vi "Compiled.Get Data Settings.vi"(6 "Cluster":refnum<k21>, 8 "error in (no error)":errorcluster, 9 "Node.Settings":T3 {"Name" format="%.0x"}, 10 "Node Ref in":T1 format="%.0x", 11 "Addon Ref In":T1 format="%.0x") -> (0 "error out":errorcluster, 1 "Node Data Refs":T4 {"Outgoing"."Trigger.Refs"."Data Reference" format="%.0x"; "Outgoing"."Disable.Refs"."Data Reference" format="%.0x"; "Outgoing"."Data.Refs"."Data Reference" format="%.0x"; "Incoming"."Timing.Refs"."Data Reference" format="%.0x"; "Incoming"."Data.Refs"."Data Reference" format="%.0x"}, 2 "Node Ref out":T1 format="%.0x", 3 "Addon Ref out":T1 format="%.0x", 4 "Async Refs":T2(array[cluster]) {"VS Refs" format="%.0x"})   [LabVIEW 2015, in "J1939 Addon System Explorer.lvlib"]
uses:
  J1939 Addon System Explorer.lvlib
  Shared/Types/Device Settings.ctl
  Shared/Types/Incoming Settings.ctl
  Shared/Types/Incoming Frame Settings.ctl
  <vilib>/NI Veristand/Custom Device API/Block Data Reference.ctl
  <vilib>/NI Veristand/Custom Device API/Data Reference.ctl
  Shared/Types/Outgoing Settings.ctl
  Shared/Types/Outgoing Frame Settings.ctl
  Shared/Types/Outgoing Event Trigger Types.ctl
  Protection Support/Source/Shared/Types/Exported Frame Settings.ctl
  Protection Support/Source/Shared/Types/Exported Frame Type.ctl
  Protection Support/Source/Shared/Types/Exported Protection Settings.ctl
  Protection Support/Source/Shared/Types/Protection Type.ctl
  Protection Support/Source/Shared/Types/XNET Signal Configuration.ctl
  Protection Support/Source/Shared/Types/Exported Counter Settings.ctl
  Protection Support/Source/Shared/Types/Exported Event Trigger Type.ctl
  <vilib>/NI Veristand/Custom Device API/Custom Device Item Ref.ctl
  Shared/Types/Monitor Settings.ctl
  <vilib>/NI Veristand/Custom Device API/Data Access Type.ctl
  Types/Compiled Refs.ctl
  Protection Support/Source/System Explorer/Types/Export Frame GUIDs List.ctl
  Protection Support/Source/System Explorer/Types/Export Frames List and Type.ctl
  Protection Support/Source/System Explorer/Types/Exported Frame Settings.ctl
  <vilib>/NI Veristand/Custom Device Tools/Custom Device Utility Library/NI VeriStand - Search for Item by GUID.vi
  Shared/SubVIs/Constants.vi
  <vilib>/NI VeriStand/Custom Device Tools/Custom Device Utility Library/Custom Device Utility Library.lvlib
  Shared/J1939 Addon Shared.lvlib
  <vilib>/NI VeriStand/Custom Device API/Custom Device API.lvlib
  Protection Support/Source/Shared/Protection and Counter Support Shared.lvlib
  Protection Support/Source/System Explorer/Protection and Counter Support System Explorer.lvlib
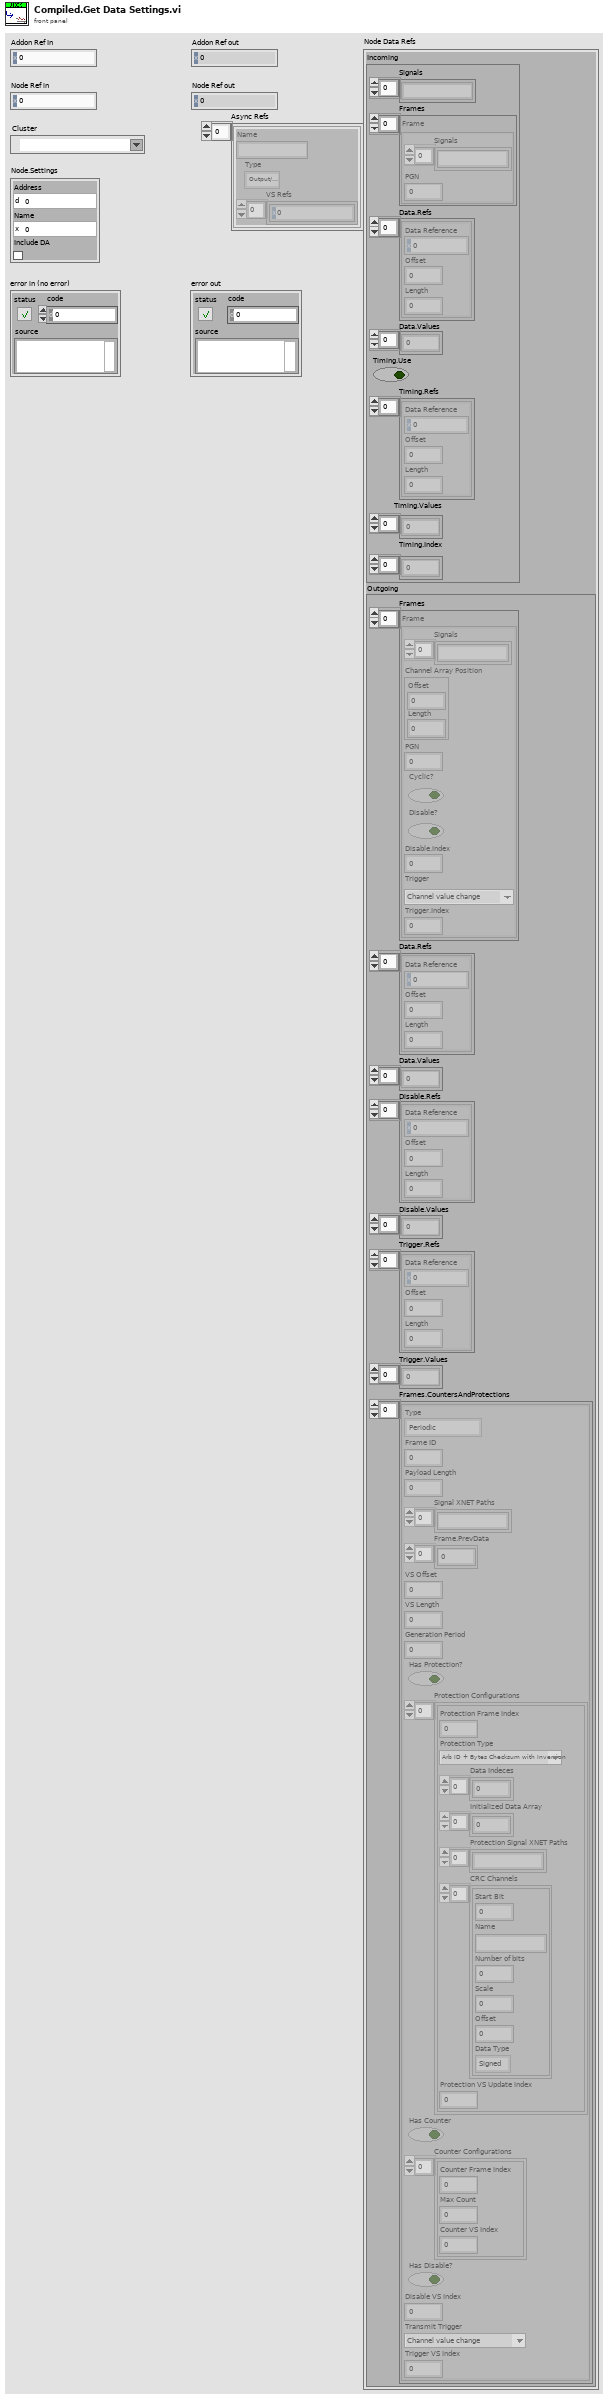
[diagram p1: front panel]
types:
  T1 = typedef "Custom Device API.lvlib/Custom Device Item Ref.ctl" = u64
  T2 = cluster{"Name":string, "Type":enum16{"Output/Write", "Input/Read", "Input/ReadWrite"}, "VS Refs":T1[]}[]
  T3 = typedef "J1939 Addon Shared.lvlib/Monitor Settings.ctl" = cluster{"Address":u8, "Name":u64, "Include DA":bool}
  T4 = typedef "J1939 Addon Shared.lvlib/Device Settings.ctl" = cluster{"Incoming":T5, "Outgoing":T9}
  T5 = typedef "J1939 Addon Shared.lvlib/Incoming Settings.ctl" = cluster{"Signals":string[], "Frames":T6[], "Data.Refs":T7[], "Data.Values":dbl[], "Timing.Use":bool, "Timing.Refs":T7[], "Timing.Values":dbl[], "Timing.Index":i32[]}
  T6 = typedef "J1939 Addon Shared.lvlib/Incoming Frame Settings.ctl" = cluster{"Signals":string[], "PGN":u32}
  T7 = typedef "Custom Device API.lvlib/Block Data Reference.ctl" = cluster{"Data Reference":T8, "Offset":u64, "Length":u64}
  T8 = typedef "Custom Device API.lvlib/Data Reference.ctl" = i32
  T9 = typedef "J1939 Addon Shared.lvlib/Outgoing Settings.ctl" = cluster{"Frames":T10[], "Data.Refs":T7[], "Data.Values":dbl[], "Disable.Refs":T7[], "Disable.Values":dbl[], "Trigger.Refs":T7[], "Trigger.Values":dbl[], "Frames.CountersAndProtections":T12[]}
  T10 = typedef "J1939 Addon Shared.lvlib/Outgoing Frame Settings.ctl" = cluster{"Signals":string[], "Channel Array Position":cluster{"Offset":u32, "Length":u32}, "PGN":u32, "Cyclic?":bool, "Disable?":bool, "Disable.Index":i32, "Trigger":T11, "Trigger.Index":i32}
  T11 = typedef "J1939 Addon Shared.lvlib/Outgoing Event Trigger Types.ctl" = enum16{"Channel value change", "Trigger channel (not zero)", "Channel value change or trigger channel (not zero)", "Trigger channel (any value change)", "Channel value change or trigger channel (any value change)"}
  T12 = typedef "Protection and Counter Support Shared.lvlib/Exported Frame Settings.ctl" = cluster{"Type":T13, "Frame ID":u32, "Payload Length":u32, "Signal XNET Paths":string[], "Frame.PrevData":dbl[], "VS Offset":i32, "VS Length":i32, "Generation Period":u32, "Has Protection?":bool, "Protection Configurations":T14[], "Has Counter":bool, "Counter Configurations":T17[], "Has Disable?":bool, "Disable VS Index":i32, "Transmit Trigger":T18, "Trigger VS Index":i32}
  T13 = typedef "Protection and Counter Support Shared.lvlib/Exported Frame Type.ctl" = enum16{"Periodic", "Event", "Periodic/Event"}
  T14 = typedef "Protection and Counter Support Shared.lvlib/Exported Protection Settings.ctl" = cluster{"Protection Frame Index":i32, "Protection Type":T15, "Data Indeces":i32[], "Initialized Data Array":dbl[], "Protection Signal XNET Paths":string[], "CRC Channels":T16[], "Protection VS Update Index":i32}
  T15 = typedef "Protection and Counter Support Shared.lvlib/Protection Type.ctl" = enum16{"Arb ID + Bytes Checksum with Inversion", "Arb ID + Bytes CRC with Inversion", "Reversed Raw Signal Checksum with Inversion"}
  T16 = typedef "Protection and Counter Support Shared.lvlib/XNET Signal Configuration.ctl" = cluster{"Start Bit":i32, "Name":string, "Number of bits":i32, "Scale":dbl, "Offset":dbl, "Data Type":u32}
  T17 = typedef "Protection and Counter Support Shared.lvlib/Exported Counter Settings.ctl" = cluster{"Counter Frame Index":i32, "Max Count":dbl, "Counter VS Index":i32}
  T18 = typedef "Protection and Counter Support Shared.lvlib/Exported Event Trigger Type.ctl" = enum16{"Channel value change", "Trigger channel (not zero)", "Channel value change or trigger channel (not zero)", "Trigger channel (any value change)", "Channel value change or trigger channel (any value change)"}
  T19 = cluster{"Name":string, "Type":enum16{"Output/Write", "Input/Read", "Input/ReadWrite"}, "VS Refs":T1[]}
  T20 = typedef "Protection and Counter Support System Explorer.lvlib/Export Frame GUIDs List.ctl" = cluster{"Signal Page GUID":string, "Rolling Counter Value GUID":string, "Protection Value GUID":string}
  T21 = typedef "J1939 Addon System Explorer.lvlib/Compiled Refs.ctl" = cluster{"VS Refs":T1[], "Disable Refs":T1[], "Trigger Refs":T1[]}
  T22 = typedef "Custom Device API.lvlib/Data Access Type.ctl" = enum16{"Read", "Write"}
  T23 = typedef "Protection and Counter Support System Explorer.lvlib/Export Frames List and Type.ctl" = cluster{"Type":T13, "Frame Refs":T1[], "Frame Settings":T24[]}
  T24 = typedef "Protection and Counter Support System Explorer.lvlib/Exported Frame Settings.ctl" = cluster{"ID":u32, "Disable Transmission":bool, "Disable Transmission Ref":T1, "Transmit Trigger":T18, "Transmit Trigger Ref":T1}
  T25 = typedef "J1939 Addon Shared.lvlib/Frame.Settings.ctl" = cluster{"ID":u32, "Disable Transmission":bool, "Disable Transmission Ref":T1, "Transmit Trigger":T11, "Transmit Trigger Ref":T1}
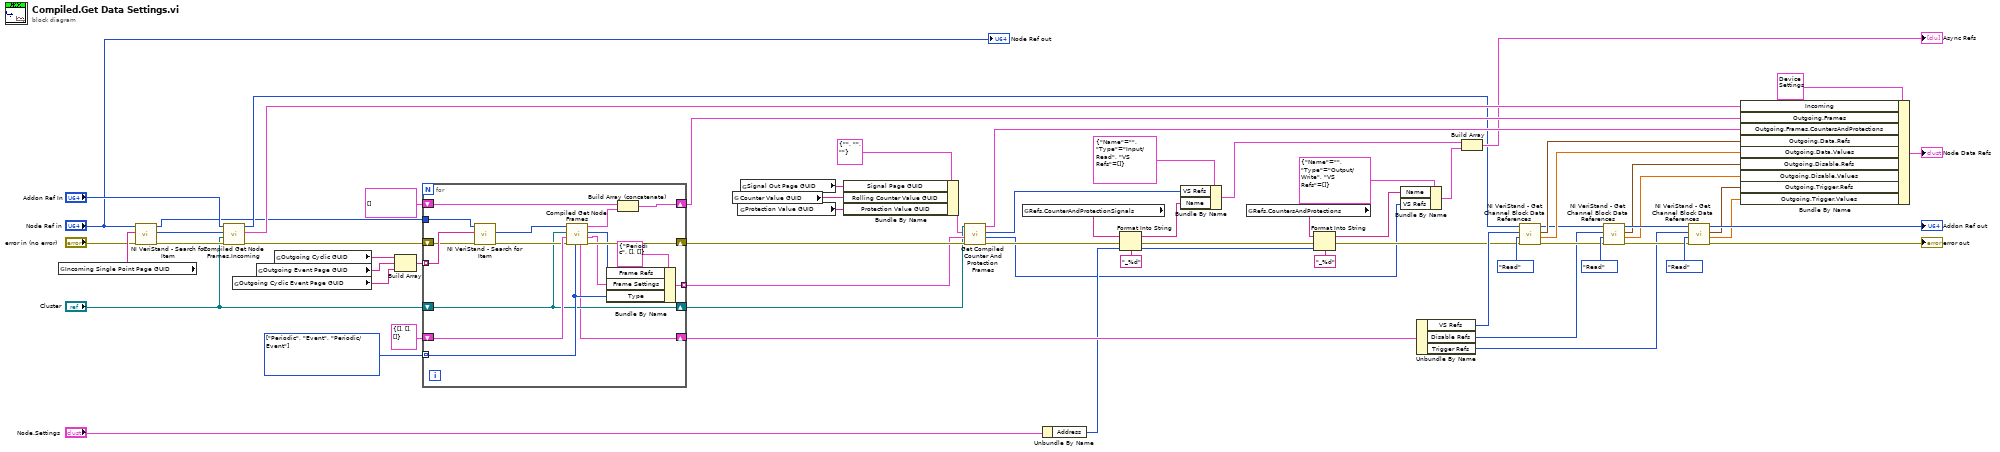
[diagram p0: block diagram]
diagram:
  w37 = T13[] [enum."Periodic", enum."Event", enum."Periodic/Event"] items=["Periodic", "Event", "Periodic/Event"]
  n1 = global read "Constants.vi" "Incoming Single Point Page GUID"() -> (w62:string)
  n2 = call-poly <vilib>:"NI VeriStand - Search for Item.vi"("error in"="error in (no error)", "Item GUID"=w62, "Section Ref in"="Node Ref in") -> ("error out"=w59:errorcluster, "Item Ref"=w60:T1, "Section Ref out"=w4:T1)  [unwired: 5 in, 1 out]
  n3 = call "Compiled Get Node Frames.Incoming.vi"("error in (no error)"=w59, "Cluster"="Cluster", "Section Ref in"=w60, "Device Ref in"="Addon Ref In") -> ("error out"=w25:errorcluster, "Incoming.Settings"=w57:T5, "Device Ref out"=w5:T1)  [unwired: 5 in]
  n4 = global read "Constants.vi" "Outgoing Cyclic Event Page GUID"() -> (w39:string)
  n5 = global read "Constants.vi" "Outgoing Event Page GUID"() -> (w40:string)
  n6 = global read "Constants.vi" "Outgoing Cyclic GUID"() -> (w41:string)
  n7 = Build Array(w41, w40, w39) -> (w38:string[])
  n8 = for {
    tunnel: w38 -> [w84] mode=indexing
    tunnel: w37 -> [w75] mode=indexing
    shift-right: [w69] -> w26
    shift-left: T21 {"VS Refs"=[], "Disable Refs"=[], "Trigger Refs"=[]} ("Refs out") -> [w82]
    shift-right: [w81] -> w34
    shift-left: w25 -> [w80]
    shift-right: [w78] -> w28
    shift-left: T10[] [] -> [w77]
    tunnel: [w73] -> w33 mode=indexing
    shift-right: [w70] -> w24
    shift-left: "Cluster" -> [w70]
    tunnel: w4 -> [w72]
    n9 = call-poly <vilib>:"NI VeriStand - Search for Item.vi"("error in"=w80, "Item GUID"=w84, "Section Ref in"=w72) -> ("error out"=w71:errorcluster, "Item Ref"=w83:T1)  [unwired: 5 in, 2 out]
    n10 = call "Compiled Get Node Frames.vi"("Type"=w75, "error in (no error)"=w71, "Refs in"=w82, "Cluster"=w70, "Section Ref in"=w83) -> ("error out"=w81:errorcluster, "Counter and Protection Frames Properties"=w68:T25[], "Counter and Protection Frames"=w74:T1[], "Standard Frames"=w79:T10[], "Refs out"=w69:T21)  [unwired: 2 in]
    n11 = Bundle By Name(cluster=T23 {"Type"=enum."Periodic", "Frame Refs"=[], "Frame Settings"=[]}, "Frame Refs"=w74, "Frame Settings"=w68, "Type"=w75) -> (w73:T23)
    n12 = Build Array (concatenate)(w77, w79) -> (w78:T10[])
  }
  n13 = global read "Constants.vi" "Counter Value GUID"() -> (w30:string)
  n14 = global read "Constants.vi" "Protection Value GUID"() -> (w29:string)
  n15 = global read "Constants.vi" "Signal Out Page GUID"() -> (w31:string)
  n16 = Bundle By Name(cluster=T20 {"Signal Page GUID"="", "Rolling Counter Value GUID"="", "Protection Value GUID"=""} ("GUIDs"), "Signal Page GUID"=w31, "Rolling Counter Value GUID"=w30, "Protection Value GUID"=w29) -> (w1:T20)
  n17 = call "Get Compiled Counter And Protection Frames.vi"("error in (no error)"=w34, "Frames per type"=w33, "GUIDs"=w1, "XNET Cluster"=w24) -> ("error out"=w16:errorcluster, "Counters and Protection Refs"=w9:T1[], "Signals Refs"=w12:T1[], "Frames"=w27:T12[])  [unwired: 4 in]
  n18 = global read "Constants.vi" "Refs.CounterAndProtectionSignals"() -> (w21:string)
  n19 = Unbundle By Name("Node.Settings") -> ("Address"=w17:u8)
  n20 = Format Into String(format string="_%d", initial string=w21, error in=w16, w17) -> (resulting string=w13:string, error out=w19:errorcluster)
  n21 = Bundle By Name(cluster=T19 {"Name"="", "Type"=enum."Input/Read", "VS Refs"=[]} ("Group"), "VS Refs"=w12, "Name"=w13) -> (w8:T19)
  n22 = global read "Constants.vi" "Refs.CountersAndProtections"() -> (w18:string)
  n23 = Format Into String(format string="_%d", initial string=w18, error in=w19, w17) -> (resulting string=w10:string, error out=w15:errorcluster)
  n24 = Bundle By Name(cluster=T19 {"Name"="", "Type"=enum."Output/Write", "VS Refs"=[]} ("Group"), "Name"=w10, "VS Refs"=w9) -> (w7:T19)
  n25 = Unbundle By Name(w26) -> ("VS Refs"=w48:T1[], "Disable Refs"=w47:T1[], "Trigger Refs"=w46:T1[])
  n26 = Build Array(w8, w7) -> (→"Async Refs":T2)
  n27 = call <vilib>:"NI VeriStand - Get Channel Block Data References.vi"("error in (no error)"=w15, "Access"=Data_Access_Type."Read", "Channel Refs"=w48, "Device Ref in"=w5) -> ("error out"=w54:errorcluster, "Values Array"=w65:dbl[], "Block Data Refs"=w64:T7[], "Device Ref out"=w50:T1)  [unwired: 4 in]
  n28 = call <vilib>:"NI VeriStand - Get Channel Block Data References.vi"("error in (no error)"=w54, "Access"=Data_Access_Type."Read", "Channel Refs"=w47, "Device Ref in"=w50) -> ("error out"=w53:errorcluster, "Values Array"=w43:dbl[], "Block Data Refs"=w42:T7[], "Device Ref out"=w51:T1)  [unwired: 4 in]
  n29 = call <vilib>:"NI VeriStand - Get Channel Block Data References.vi"("error in (no error)"=w53, "Access"=Data_Access_Type."Read", "Channel Refs"=w46, "Device Ref in"=w51) -> ("error out"=→"error out":errorcluster, "Values Array"=w45:dbl[], "Block Data Refs"=w44:T7[], "Device Ref out"=→"Addon Ref out":T1)  [unwired: 4 in]
  n30 = Bundle By Name(cluster=T4 {"Incoming"={"Signals"=[], "Frames"=[], "Data.Refs"=[], "Data.Values"=[], "Timing.Use"=FALSE, "Timing.Refs"=[], "Timing.Values"=[], "Timing.Index"=[]}, "Outgoing"={"Frames"=[], "Data.Refs"=[], "Data.Values"=[], "Disable.Refs"=[], "Disable.Values"=[], "Trigger.Refs"=[], "Trigger.Values"=[], "Frames.CountersAndProtections"=[]}} ("Data"), "Incoming"=w57, "Outgoing.Frames"=w28, "Outgoing.Frames.CountersAndProtections"=w27, "Outgoing.Data.Refs"=w64, "Outgoing.Data.Values"=w65, "Outgoing.Disable.Refs"=w42, "Outgoing.Disable.Values"=w43, "Outgoing.Trigger.Refs"=w44, "Outgoing.Trigger.Values"=w45) -> (→"Node Data Refs":T4)
  "Node Ref out" <- "Node Ref in"
